vi "mlink_ao_scan.vi"(8 "error in (no error)":errorcluster, 11 "connection ID":i32=-1) -> (0 "error out":errorcluster, 3 "connection ID out":i32)   [LabVIEW 2009, in "MicroDAQ.lvlib" / "mlink.lvlib"]
doc: "This function starts analog output scanning. A function call has to be preceded with mlink_ao_scan_init() which initiates analog output scanning session parameters. Function \nenables MicroDAQ hardware to output data on selected AO channels. In order to stop \nscanning, function mlink_ao_scan_stop() has to be called."
uses:
  <instrlib>/MicroDAQ/Mlink library wraper/mlink.lvlib
  <instrlib>/MicroDAQ/MLink32.dll
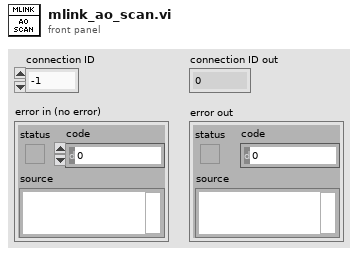
[diagram p1: front panel]
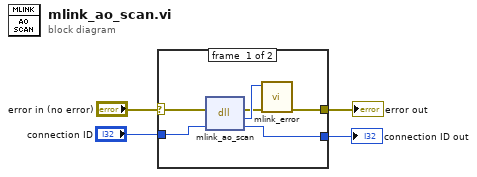
[diagram p0: block diagram]
diagram:
  n1 = case shown="No Error" "error in (no error)" {
    selector: "error in (no error)" -> [w10 w11]
    tunnel: [w9 w12] -> w3
    tunnel: "connection ID" -> [w8 w12]
    tunnel: [w5 w11] -> w1
    frame #0 {
      n2 = dll-call lib="C:/Program Files (x86)/National Instruments/LabVIEW 2009/instr.lib/MicroDAQ/MLink32.dll" fn="mlink_ao_scan"(error in=w10, "connection ID"=w8) -> (error out=w6:errorcluster, "return type"=w7:i32, "connection ID"=w9:i32)  [unwired: 2 in, 1 out]
      n3 = call <instrlib>:"mlink_error.vi"("error in (no error)"=w6, "error code"=w7) -> ("error out"=w5:errorcluster)  [unwired: 9 in]
    }
    frame #1 {
    }
  }
  "connection ID out" <- w3
  "error out" <- w1
